vi "open.vi"(8 "error in (no error)":errorcluster caption="错误输入（无错误）", 10 "index (row)":i8=75, 11 "LXMCU_40G 输入":refnum<class "LXMCU_40G.lvclass"> caption="DNL_LabVIEW Object in") -> (0 "error out":errorcluster caption="错误输出", 3 "LXMCU_40G 输出":refnum<class "LXMCU_40G.lvclass"> caption="DNL_LabVIEW Object out")   [LabVIEW 2011, in "LXMCU_40G.lvclass"]
uses:
  LXMCU_40G.lvclass
  LXMCU_40G.lvclass/LXMCU_40G.ctl
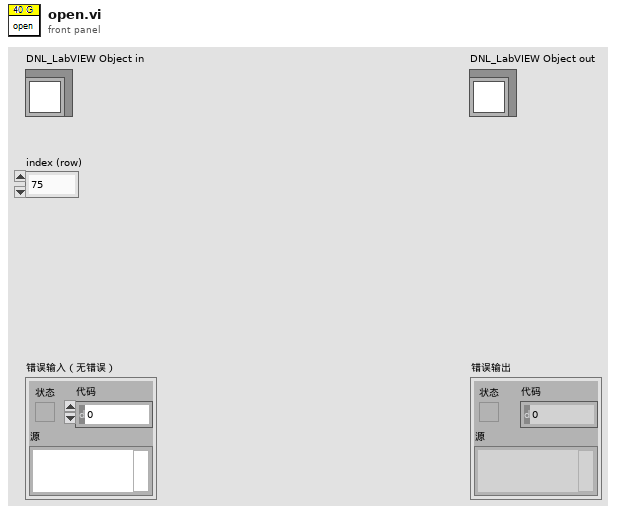
[diagram p1: front panel]
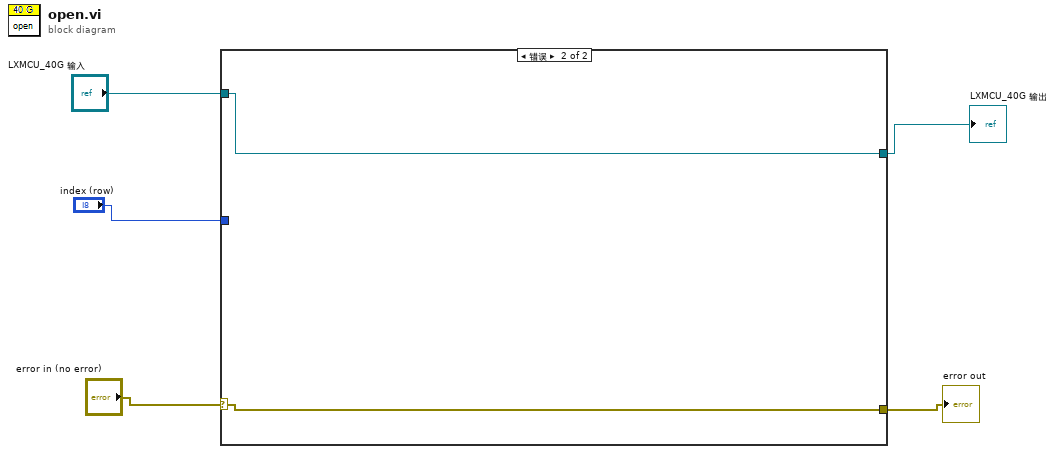
[diagram p0: block diagram]
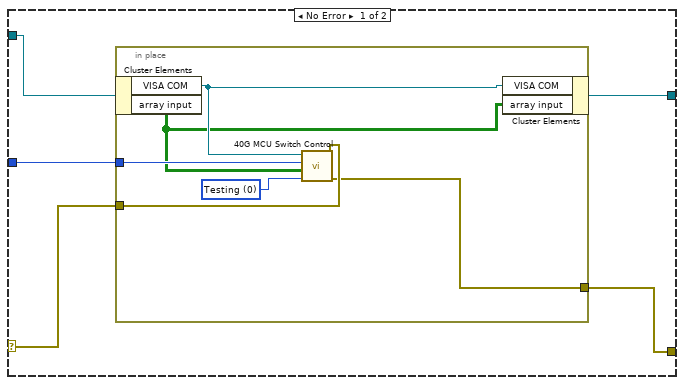
[diagram p2: hidden frame]
diagram:
  n1 = case shown="错误" "error in (no error)" {
    selector: "error in (no error)" -> [w8 w17]
    tunnel: "LXMCU_40G 输入" -> [w10 w18]
    tunnel: "index (row)" -> [w9 _]
    tunnel: [w7 w17] -> w2
    tunnel: [w6 w18] -> w1
    frame No Error {
      n2 = in-place {
        in-place-border: w9 -> [w16]
        in-place-border: w8 -> [w14]
        in-place-border: [w13] -> w7
        w15 = u16 0 items=["Testing", "Close All"] ("Function")
        n3 = in-place-cluster #1(w10) -> ("VISA COM"=w12:refnum<visa-resource-name>, "array input"=w11:bool[][])
        n4 = call "40G MCU Switch Control.vi"("Error in"=w14, "Function"=w15, "Array input:"=w11, "Index"=w16, "VISA"=w12) -> ("error out"=w13:errorcluster)  [unwired: 6 in]
        n5 = in-place-cluster #1("VISA COM"=w12, "array input"=w11) -> (w6:refnum<class "LXMCU_40G.lvclass">)
      }
    }
    frame Error {
    }
  }
  "error out" <- w2
  "LXMCU_40G 输出" <- w1
